vi "SVT Get Spectrum Value (1 Ch).vi"(0 "spectrum":cluster{"x0":dbl, "dx":dbl, "magnitude":dbl[]} {"magnitude" format="%.2f"; "dx" format="%.2f"; "x0" format="%.2f"}, 2 "frequency [Hz]":dbl=1000.0 format="%.2f", 3 "frequency coercion":T1(ring), 4 "spectrum info":T2={"channel name"="", "description"="", "x-axis units"=0, "spectral info"={"spectrum type"=enum."Power [Magnitude^2]", "linear/dB"=enum."linear", "window"=0, "window size"=0, "FFT size"=0}, "engineering units"=0, "custom label"="", "dB reference [EU]"=0.0, "peak units"=enum."rms", "weighting filter"=0, "spectral density?"=FALSE, "unit label"="", "spectrum skewed?"=FALSE, "complimentary spectrum units"=enum."none"} {"x-axis units" items=["Time (s)"=0, "Frequency-CB (Hz)"=1, "Frequency-CPB (Hz)"=1248, "Frequency-Arbitrary (Hz)"=2357, "Quefrency (s)"=2, "Revolutions (rev)"=3, "Order"=4, "Speed (RPM)"=11, "Speed (rad/s)"=21, "Index"=65535]; "weighting filter" items=["Linear", "A-weighting", "B-weighting", "C-weighting", "ITU-R 468-4", "Dolby", "CCITT", "C-message", "Wb", "Wc", "Wd", "We", "Wf", "Wh", "Wj", "Wk", "Wm", "AES17 20 kHz lowpass", "AES17 40 kHz lowpass", "AES17 20 kHz highpass", "AES17 40 kHz highpass"]; "dB reference [EU]" format="%.2f"; "engineering units" items=["custom..."=0, "V"=1, "A"=21, "C"=30, "pC"=31, "s"=32, "-"=29, "Pa"=2, "N"=20, "g"=3, "m/s^2"=4, "m/s"=5, "m"=6, "mm/s"=12, "mm"=13, "micron/s"=14, "micron"=15, "in/s^2"=7, "in/s"=8, "in"=9, "mil/s"=10, "mil"=11, "rad/s^2"=16, "rad/s"=17, "rad"=18, "deg/s^2"=26, "deg/s"=27, "deg"=28, "RPM"=22, "cycle/s^2"=23, "Hz"=24, "cycle"=25, "strain"=19]; "spectral info"."window" items=["None "=0, "Hanning"=1, "Hamming"=2, "Blackman-Harris"=3, "Exact Blackman"=4, "Blackman"=5, "Flat Top"=6, "4 Term B-Harris "=7, "7 Term B-Harris"=8, "Low Sidelobe"=9, "Force - Exponential"=10, "Gaussian"=62]}, 5 "error in (no error)":errorcluster) -> (14 "spectrum value":dbl=nan format="%.2p", 15 "unit label":string, 16 "actual frequency [Hz]":dbl=nan format="%.2f", 17 "frequency label":string, 19 "error out":errorcluster)   [LabVIEW 2017]
doc: "Extracts the value of the spectrum at the specified frequency. Use the frequency coercion control to specify how the frequency should be coerced if it does not exactly coincide with a frequency line. This VI operates on any real-valued spectrum."
uses:
  <vilib>/addons/_NISVFA/_Shared subVIs/Controls/svc_Spectrum Info.ctl
  <vilib>/addons/_NISVFA/_Shared subVIs/Controls/svc_X-Axis Units.ctl
  <vilib>/addons/_NISVFA/_Shared subVIs/Controls/svc_Spectrum Type.ctl
  <vilib>/addons/_NISVFA/_Shared subVIs/Controls/svc_Engineering Units Text Ring.ctl
  <vilib>/addons/_NISVFA/_Shared subVIs/Controls/svc_Weighting Filter Text Ring.ctl
  <vilib>/addons/_NISVFA/_Shared subVIs/Controls/svc_Complimentary Spectrum Units.ctl
  <vilib>/addons/_NISVFA/_Shared subVIs/Common/svc_Get Weighting Enum and Labels.vi
  <vilib>/addons/_NISVFA/_Shared subVIs/Common/svc_Unit Label Lexical Class.vi
  <vilib>/addons/_NISVFA/_Shared subVIs/Common/svc_Engineering Units to Unit Label.vi
  <vilib>/addons/_NISVFA/_Shared subVIs/Common/svc_Format Value (DBL).vi
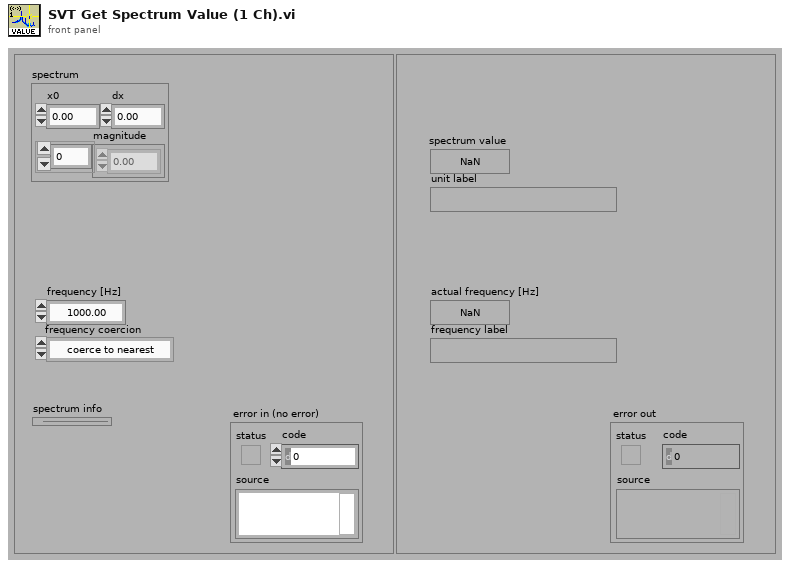
[diagram p1: front panel]
types:
  T1 = enum16{"coerce to nearest", "coerce to next highest", "coerce to next lowest", "interpolate"}
  T2 = typedef "svc_Spectrum Info.ctl" = cluster{"channel name":string, "description":string, "x-axis units":T3, "spectral info":cluster{"spectrum type":T4, "linear/dB":enum16{"linear", "dB"}, "window":u16, "window size":i32, "FFT size":i32}, "engineering units":T5, "custom label":string, "dB reference [EU]":dbl, "peak units":enum16{"rms", "peak", "peak-peak"}, "weighting filter":T6, "spectral density?":bool, "unit label":string, "spectrum skewed?":bool, "complimentary spectrum units":T7}
  T3 = typedef "svc_X-Axis Units.ctl" = u16
  T4 = typedef "svc_Spectrum Type.ctl" = enum16{"FFT Spectrum [complex]", "Amplitude [Magnitude]", "Power [Magnitude^2]", "Cross Spectrum [complex]", "Frequency Response [Complex]"}
  T5 = typedef "svc_Engineering Units Text Ring.ctl" = u16
  T6 = typedef "svc_Weighting Filter Text Ring.ctl" = u16
  T7 = typedef "svc_Complimentary Spectrum Units.ctl" = enum16{"none", "radians", "degrees", "cycles", "imaginary"}
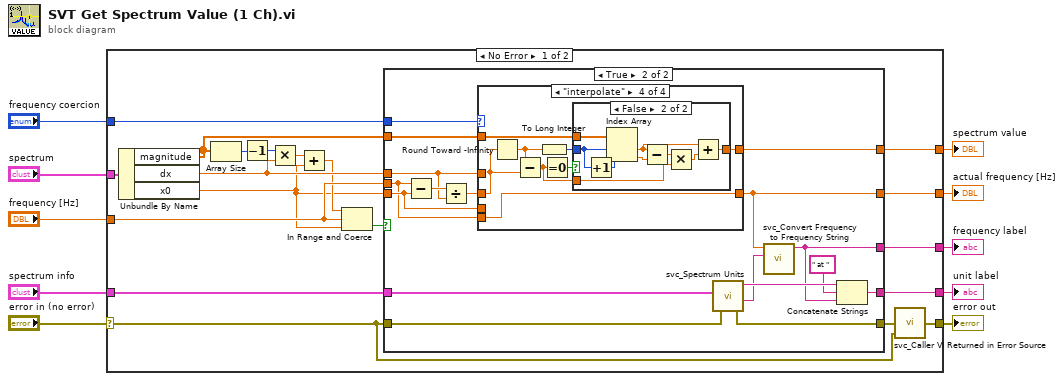
[diagram p0: block diagram]
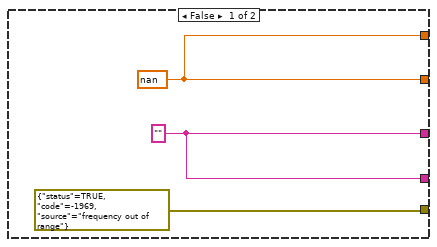
[diagram p2: hidden frame]
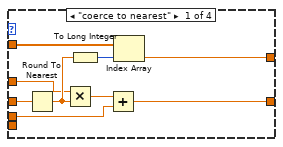
[diagram p3: hidden frame]
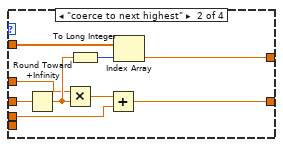
[diagram p4: hidden frame]
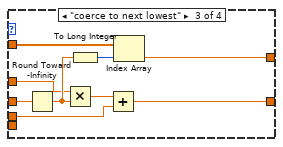
[diagram p5: hidden frame]
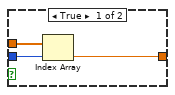
[diagram p6: hidden frame]
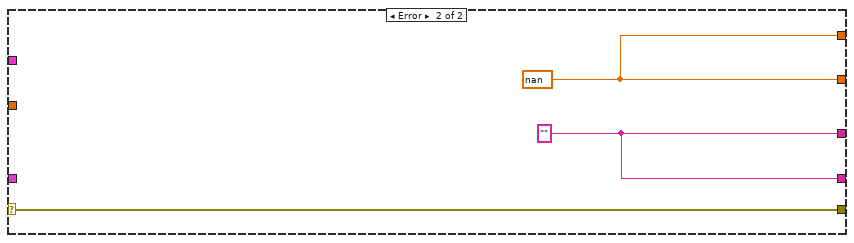
[diagram p7: hidden frame]
diagram:
  n1 = case shown="No Error" "error in (no error)" {
    selector: "error in (no error)" -> [w11 w99]
    tunnel: [w13 w99] -> w10
    tunnel: "spectrum" -> [w29 _]
    tunnel: [w27 w97] -> w8
    tunnel: "spectrum info" -> [w28 _]
    tunnel: "frequency coercion" -> [w21 _]
    tunnel: "frequency [Hz]" -> [w18 _]
    tunnel: [w24 w98] -> w4
    tunnel: [w23 w98] -> w3
    tunnel: [w20 w97] -> w2
    frame No Error {
      n2 = Unbundle By Name(w29) -> ("magnitude"=w17:dbl[], "dx"=w22:dbl, "x0"=w14:dbl)
      n3 = Array Size(array=w17) -> (size(s)=w26:i32)
      n4 = Decrement(x=w26) -> (x-1=w25:i32)
      n5 = Multiply(x=w25, y=w22) -> (x*y=w16:dbl)
      n6 = Add(x=w16, y=w14) -> (x+y=w15:dbl)
      n7 = In Range and Coerce(upper limit=w15, x=w18, lower limit=w14) -> (In Range?=w19:bool)  [unwired: 1 out]
      n8 = case shown="True" w19 {
        tunnel: w28 -> [_ w49]
        tunnel: w11 -> [_ w48]
        tunnel: [errorcluster {"status"=TRUE, "code"=-1969, "source"="frequency out of range"} ("error out") w47] -> w12
        tunnel: w17 -> [_ w46]
        tunnel: [w30 w44] -> w27
        tunnel: [w31 w36] -> w24
        tunnel: [w31 w37] -> w23
        tunnel: w18 -> [_ w35]
        tunnel: w14 -> [_ w38]
        tunnel: w22 -> [_ w39]
        tunnel: w21 -> [_ w41]
        tunnel: [w30 w34] -> w20
        frame False {
          w30 = ""
          w31 = nan ("frequency [Hz]")
        }
        frame True {
          n9 = Subtract(x=w35, y=w38) -> (x-y=w42:dbl)
          n10 = Divide(x=w42, y=w39) -> (x/y=w40:dbl)
          n11 = case shown="\"interpolate\"" w41 {
            tunnel: w46 -> [w58 w67 w76 w84]
            tunnel: w40 -> [w57 w66 w75 w77]
            tunnel: w39 -> [w54 w63 w72 _]
            tunnel: w38 -> [w51 w60 w69 _]
            tunnel: [w53 w62 w71 w82] -> w37
            tunnel: [w52 w61 w70 w78] -> w36
            tunnel: w35 -> [_ _ _ w78]
            frame "coerce to nearest" {
              n12 = Round To Nearest(number=w57) -> (nearest integer value=w55:dbl)
              n13 = Multiply(x=w54, y=w55) -> (x*y=w50:dbl)
              n14 = To Long Integer(number=w55) -> (32bit integer=w56:i32)
              n15 = Add(x=w50, y=w51) -> (x+y=w52:dbl)
              n16 = Index Array(array=w58, index=w56) -> (element=w53:dbl)
            }
            frame "coerce to next highest" {
              n17 = Round Toward +Infinity ("Round To +Infinity")(x=w66) -> (ceil(x): smallest int >= x=w64:dbl)
              n18 = Multiply(x=w63, y=w64) -> (x*y=w59:dbl)
              n19 = To Long Integer(number=w64) -> (32bit integer=w65:i32)
              n20 = Add(x=w59, y=w60) -> (x+y=w61:dbl)
              n21 = Index Array(array=w67, index=w65) -> (element=w62:dbl)
            }
            frame "coerce to next lowest" {
              n22 = Round Toward -Infinity ("Round To -Infinity")(1:w75) -> (0:w73:dbl)
              n23 = Multiply(x=w72, y=w73) -> (x*y=w68:dbl)
              n24 = To Long Integer(number=w73) -> (32bit integer=w74:i32)
              n25 = Add(x=w68, y=w69) -> (x+y=w70:dbl)
              n26 = Index Array(array=w76, index=w74) -> (element=w71:dbl)
            }
            frame "interpolate" {
              n27 = Round Toward -Infinity ("Round To -Infinity")(1:w77) -> (0:w81:dbl)
              n28 = Subtract(x=w81, y=w77) -> (x-y=w79:dbl)
              n29 = To Long Integer(number=w81) -> (32bit integer=w83:i32)
              n30 = Equal To 0?(x=w79) -> (x = 0?=w80:bool)
              n31 = case shown="False" w80 {
                tunnel: w84 -> [w87 w96]
                tunnel: w83 -> [w86 w94]
                tunnel: [w85 w90] -> w82
                tunnel: w79 -> [_ w92]
                frame True {
                  n32 = Index Array(array=w87, index=w86) -> (element=w85:dbl)
                }
                frame False {
                  n33 = Increment(x=w94) -> (x+1=w95:i32)
                  n34 = Index Array(array=w96, index #1=w94, index #2=w95) -> (element #1=w89:dbl, element #2=w93:dbl)
                  n35 = Subtract(x=w89, y=w93) -> (x-y=w91:dbl)
                  n36 = Multiply(x=w91, y=w92) -> (x*y=w88:dbl)
                  n37 = Add(x=w89, y=w88) -> (x+y=w90:dbl)
                }
              }
            }
          }
          n38 = call <vilib>:"svc_Spectrum Units.vi"("error in (no error)"=w48, "spectrum info in"=w49) -> ("error out"=w47:errorcluster, "x-axis unit label"=w33:string, "unit label"=w45:string)  [unwired: 2 in, 1 out]
          n39 = call <vilib>:"svc_Convert Frequency to Frequency String.vi"("x-axis unit label"=w33, "frequency [Hz]"=w36) -> ("frequency string"=w34:string)  [unwired: 9 in]
          n40 = Concatenate Strings(w45, " at " ("string"), w34) -> (w44:string)
        }
      }
      n41 = call <vilib>:"svc_Caller VI Returned in Error Source.vi"("warning input to caller"=w11, "error in (no error)"=w12) -> ("error out"=w13:errorcluster)  [unwired: 3 in]
    }
    frame Error {
      w98 = nan ("frequency [Hz]")
      w97 = "" ("frequency range string")
    }
  }
  "error out" <- w10
  "unit label" <- w8
  "actual frequency [Hz]" <- w4
  "spectrum value" <- w3
  "frequency label" <- w2
